vi "Write Events.vi"(8 "error in (no error)":errorcluster, 10 "Events":T1, 11 "Recipe State Data in":refnum<class "Recipe State Data.lvclass">) -> (0 "error out":errorcluster, 3 "Recipe State Data out":refnum<class "Recipe State Data.lvclass">)   [LabVIEW 2022 SP3, in "Recipe State Data.lvclass"]
uses:
  Recipe State Data.lvclass
  Recipe State Data.lvclass/Recipe State Data.ctl
  Events.ctl
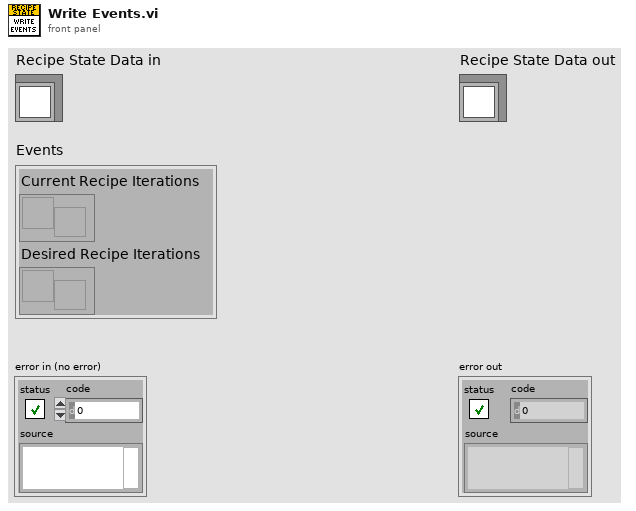
[diagram p1: front panel]
types:
  T1 = typedef "Recipe State Data.lvclass/Events.ctl" = cluster{"Current Recipe Iterations":refnum<user-event>, "Desired Recipe Iterations":refnum<user-event>}
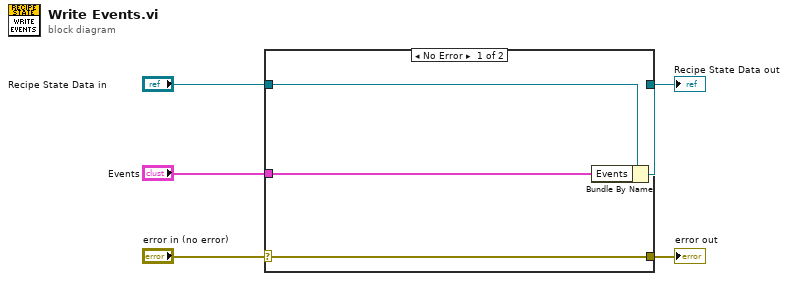
[diagram p0: block diagram]
diagram:
  n1 = case shown="No Error" "error in (no error)" {
    selector: "error in (no error)" -> [w9 w10]
    tunnel: [w9 w10] -> w4
    tunnel: [w7 w11] -> w2
    tunnel: "Recipe State Data in" -> [w8 w11]
    tunnel: "Events" -> [w6 _]
    frame No Error {
      n2 = Bundle By Name(cluster=w8, "Events"=w6) -> (w7:refnum<class "Recipe State Data.lvclass">)
    }
    frame Error {
    }
  }
  "error out" <- w4
  "Recipe State Data out" <- w2
